vi "Inst.Transport.GetPublicEvents.vi"(8 "error in (no error)":errorcluster, 11 "Inst.Transport in":refnum<class "Inst.Transport.lvclass">) -> (0 "error out":errorcluster, 2 "Transport Public Events":T1, 3 "Inst.Transport out":refnum<class "Inst.Transport.lvclass">)   [LabVIEW 2019, in "Inst.Transport.lvclass"]
uses:
  Inst.Transport.lvclass
  Typedefs/UI State--enum.ctl
  Typedefs/PublicEvents--Cluster.ctl
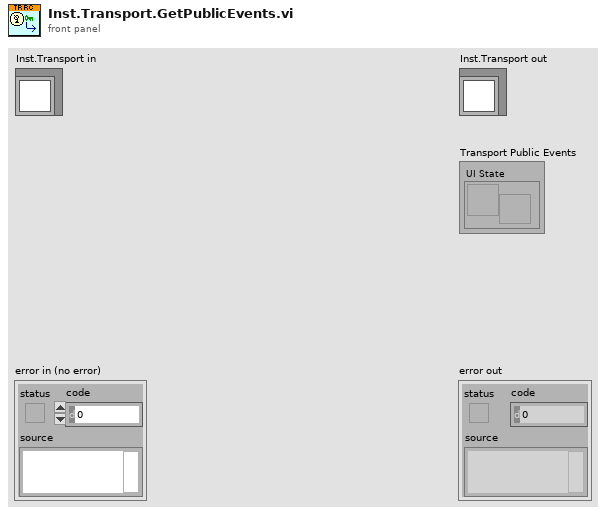
[diagram p1: front panel]
types:
  T1 = typedef "Inst.Transport.lvclass/PublicEvents--Cluster.ctl" = cluster{"UI State":refnum<user-event>}
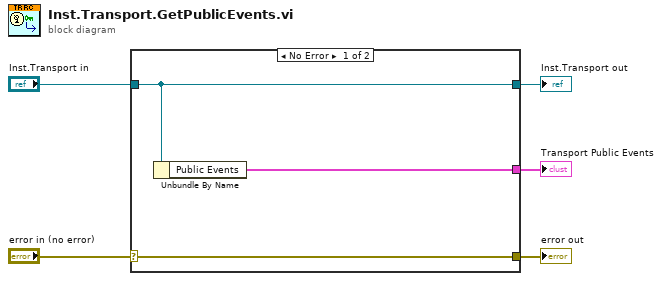
[diagram p0: block diagram]
diagram:
  n1 = case shown="No Error" "error in (no error)" {
    selector: "error in (no error)" -> [w8 w9]
    tunnel: [w8 w9] -> w4
    tunnel: [w6 w10] -> w2
    tunnel: "Inst.Transport in" -> [w6 w10]
    tunnel: [w7 _] -> w1
    frame No Error {
      n2 = Unbundle By Name(w6) -> ("Public Events"=w7:T1)
    }
    frame Error {
    }
  }
  "error out" <- w4
  "Inst.Transport out" <- w2
  "Transport Public Events" <- w1
